vi "Comm.vi"(8 "error in (no error)":errorcluster, 11 "NXP in":refnum<class "NXP.lvclass">) -> (0 "error out":errorcluster, 2 "String":string, 3 "NXP out":refnum<class "NXP.lvclass">)   [LabVIEW 2020, in "NXP.lvclass"]
uses:
  NXP.lvclass
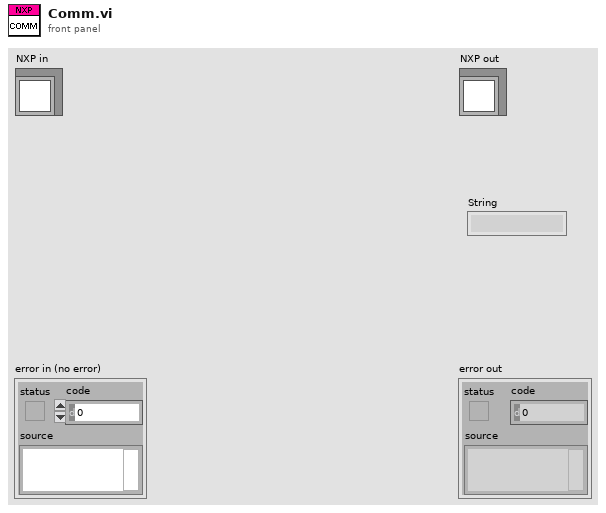
[diagram p1: front panel]
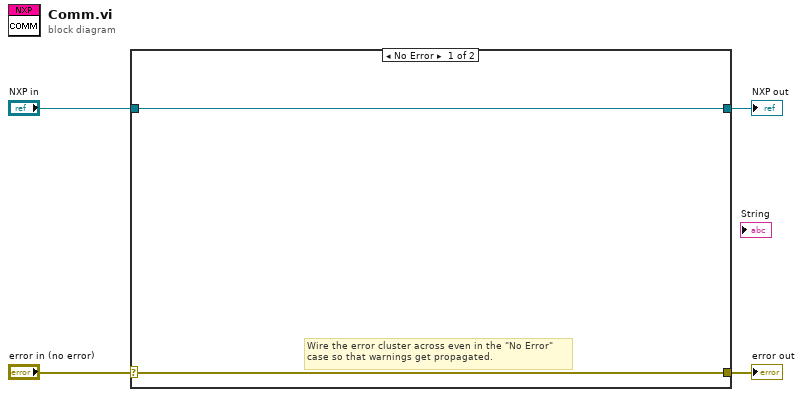
[diagram p0: block diagram]
diagram:
  n1 = case shown="No Error" "error in (no error)" {
    selector: "error in (no error)" -> [w6 w8]
    tunnel: [w6 w8] -> w3
    tunnel: [w5 w7] -> w1
    tunnel: "NXP in" -> [w5 w7]
    frame No Error {
      # "Wire the error cluster across even in the \"No Error\"\ncase so that warnings get propagated."
    }
    frame Error {
    }
  }
  "error out" <- w3
  "NXP out" <- w1
